vi "(SubVI) frame to time(s).vi"(11 "Numeric in":dbl) -> (3 "Numeric out":dbl)   [LabVIEW 2016]
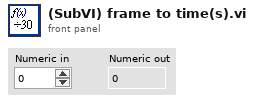
[diagram p1: front panel]
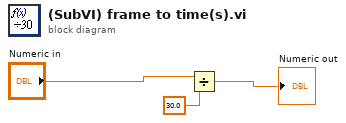
[diagram p0: block diagram]
diagram:
  n1 = Divide(x="Numeric in", y=30.0 ("x/y")) -> (x/y=→"Numeric out":dbl)
